vi "meta PID - V1.vi"(4 "default output":dbl=1.0, 6 "input parameter":dbl=300.0, 7 "control?":bool, 8 "lower limit":dbl=-inf, 9 "upper limit":dbl=inf, 10 "sweep folder path":path, 11 "ctl name dispatch":T1) -> (0 "bezier output":dbl, 1 "frequencies":dbl[](array[numeric]), 2 "temperatures":dbl[](array[numeric]), 3 "ok":bool)   [LabVIEW 2015]
uses:
  ctl -- name dispatcher -- action.ctl
  next chunk read-write PID -- action.ctl
  file -- 9w path.vi
  array -- find index - real.vi
  array -- interpolate -- i.vi
  Q - not nan -- real.vi
  <vilib>/Utility/libraryn.llb/Check if File or Folder Exists.vi
  file -- read list of lines.vi
  parse -- find first line.vi
  parse -- get list of matches -- numbers.vi
  <vilib>/Utility/file.llb/Write To Spreadsheet File.vi
  <vilib>/Utility/file.llb/Write To Spreadsheet File (string).vi
  <vilib>/gmath/function.llb/Binomial Coefficient.vi
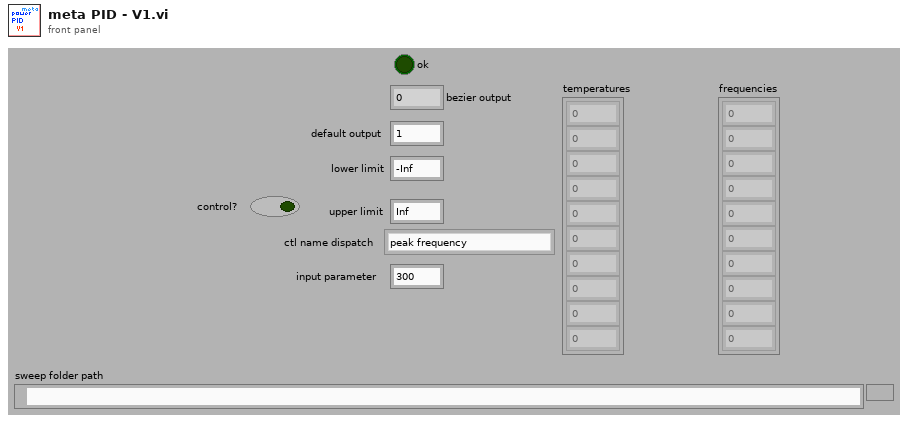
[diagram p1: front panel]
types:
  T1 = typedef "ctl -- name dispatcher -- action.ctl" = enum16{"peak frequency", "peak frequency DUMP", "peak gamma DUMP", "peak gamma", "peak frequency TEST", "peak gamma TEST", "ultrasonic power", "time in gamma", "set temperature ", "set temperature timer", "peak default gamma", "last scan file", "peak freq gamma TEST", "peak NAMES", "errors", "P_I_D", "P", "I", "D", "power vs time", "power vs time TIMER", "void", "power log", "set temperature - SINE", "itc ltc log", "peak - time in gamma"}
  T2 = typedef "next chunk read-write PID -- action.ctl" = enum16{"read", "interpolate", "append col", "write", "write PID col", "append PID col", "interpolate - bezier"}
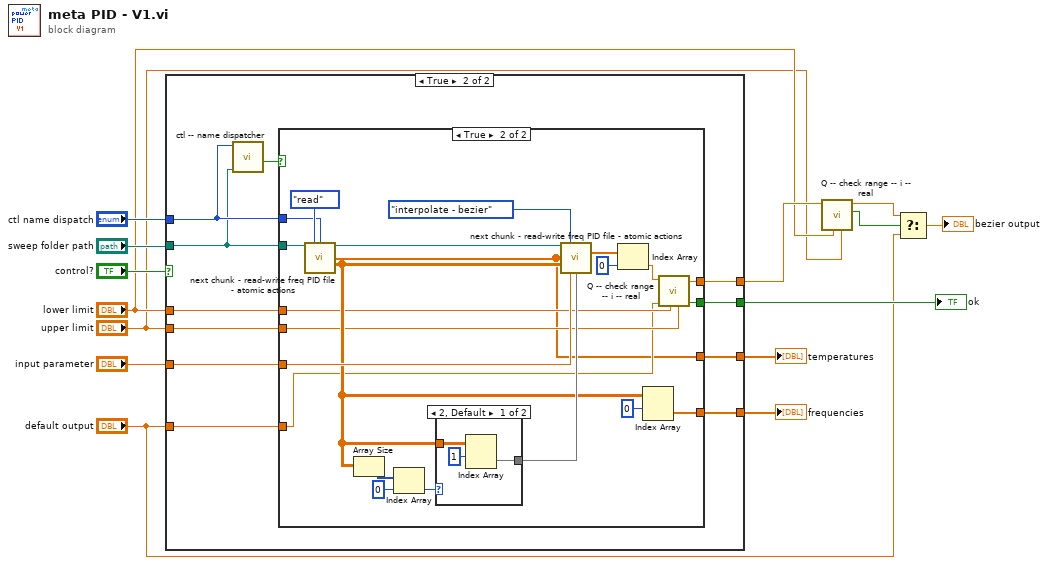
[diagram p0: block diagram]
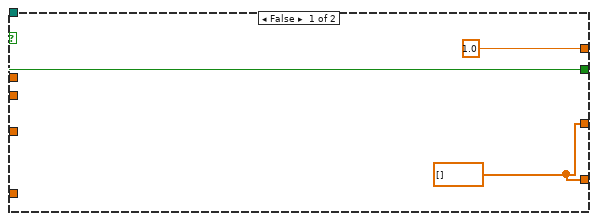
[diagram p2: hidden frame]
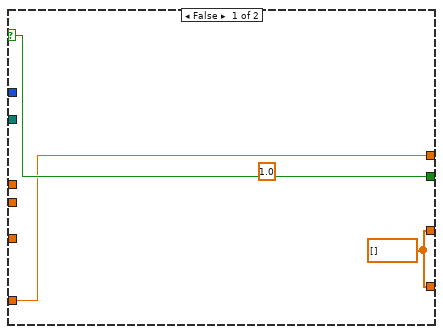
[diagram p3: hidden frame]
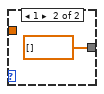
[diagram p4: hidden frame]
diagram:
  n1 = case shown="True" "control?" {
    selector: "control?" -> [w15 _]
    tunnel: "sweep folder path" -> [_ w19]
    tunnel: "input parameter" -> [_ w28]
    tunnel: [1.0 ("upper") w27] -> w7
    tunnel: [w16 w26] -> w11
    tunnel: [w16 w25] -> w10
    tunnel: "lower limit" -> [_ w24]
    tunnel: "upper limit" -> [_ w23]
    tunnel: [w15 w22] -> w9
    tunnel: "ctl name dispatch" -> [_ w20]
    tunnel: "default output" -> [_ w18]
    frame False {
      w16 = dbl[] [] ("temperatures")
    }
    frame True {
      n2 = call "ctl -- name dispatcher.vi"("sweep folder path"=w19, "ctl name dispatch"=w20) -> ("file or folder exists?"=w21:bool)  [unwired: 7 in, 2 out]
      n3 = case shown="True" w21 {
        selector: w21 -> [w30 _]
        tunnel: w19 -> [_ w50]
        tunnel: w20 -> [_ w46]
        tunnel: w28 -> [_ w49]
        tunnel: [w29 w44] -> w27
        tunnel: [w31 w32] -> w26
        tunnel: [w31 w42] -> w25
        tunnel: w24 -> [_ w36]
        tunnel: w23 -> [_ w35]
        tunnel: [w30 w34] -> w22
        tunnel: w18 -> [w29 w33]
        frame False {
          w31 = dbl[] [] ("temperatures")
          (unwired) 1.0 ("upper")
        }
        frame True {
          n4 = call "next chunk - read-write freq PID file - atomic actions .vi"("sweep folder path"=w50, "PID action"=next_chunk_read-write_PID_--_action."read", "ctl kind IN"=w46) -> ("sweep folder path out"=w52:path, "temperatures"=w32:dbl[], "frequencies"=w37:dbl[][])  [unwired: 8 in, 2 out]
          n5 = Array Size(array=w37) -> (size(s)=w41:i32[])
          n6 = Index Array(array=w41, index=0) -> (element=w39:i32)
          n7 = case shown="2, Default" w39 {
            tunnel: [w54 dbl[] []] -> w38
            tunnel: w37 -> [w56 _]
            frame 2, Default {
              n8 = Index Array(array=w56, index (row)=1) -> (element=w54:dbl[])  [unwired: 1 in]
            }
            frame 1 {
            }
          }
          n9 = call "next chunk - read-write freq PID file - atomic actions .vi"("sweep folder path"=w52, "PID action"=next_chunk_read-write_PID_--_action."interpolate - bezier", "temperatures IN"=w32, "frequencies IN"=w37, "temperature"=w49, "weights"=w38) -> ("PID freq"=w48:dbl[])  [unwired: 5 in, 4 out]
          n10 = Index Array(array=w48, index=0) -> (element=w45:dbl)
          n11 = Index Array(array=w37, index (row)=0) -> (element=w42:dbl[])  [unwired: 1 in]
          n12 = call "Q -- check range -- i -- real.vi"("upper"=w35, "lower"=w36, "default"=w33, "number"=w45) -> ("in range?"=w34:bool, "number in range"=w44:dbl)  [unwired: 5 in, 1 out]
        }
      }
    }
  }
  "temperatures" <- w11
  "frequencies" <- w10
  "ok" <- w9
  n13 = call "Q -- check range -- i -- real.vi"("upper"="upper limit", "lower"="lower limit", "number"=w7) -> ("in range?"=w4:bool, "number in range"=w3:dbl)  [unwired: 6 in, 1 out]
  n14 = Select(t=w3, s=w4, f="default output") -> (s? t:f=→"bezier output":dbl)
